vi "Send Perform Action.vi"(4 "Timeout":i32=1000, 6 "DataSocket Reply URL":string, 7 "Message Priority (Normal)":T1=enum."Normal", 8 "error in (no error)":errorcluster, 9 "Input":variant, 10 "Task-Point Ident":string, 11 "Message Enqueuer":refnum<class "Message Enqueuer.lvclass">) -> (0 "error out":errorcluster, 1 "Timeout?":bool, 2 "Reply":variant, 3 "Message Enqueuer out":refnum<class "Message Enqueuer.lvclass">)   [LabVIEW 2024, in "IMSS Target Actor.lvlib" / "Perform Action Msg.lvclass"]
doc: "This VI sends the message to an actor."
uses:
  Perform Action Msg.lvclass
  <vilib>/ActorFramework/Message Enqueuer/Message Enqueuer.lvclass
  <vilib>/ActorFramework/Message Enqueuer/Message Priority.ctl
  Perform Action Msg.lvclass/Perform Action Msg.ctl
  Reply-Msg-DataSocket/Reply Msg DataSocket/Reply Msg DataSocket.lvclass
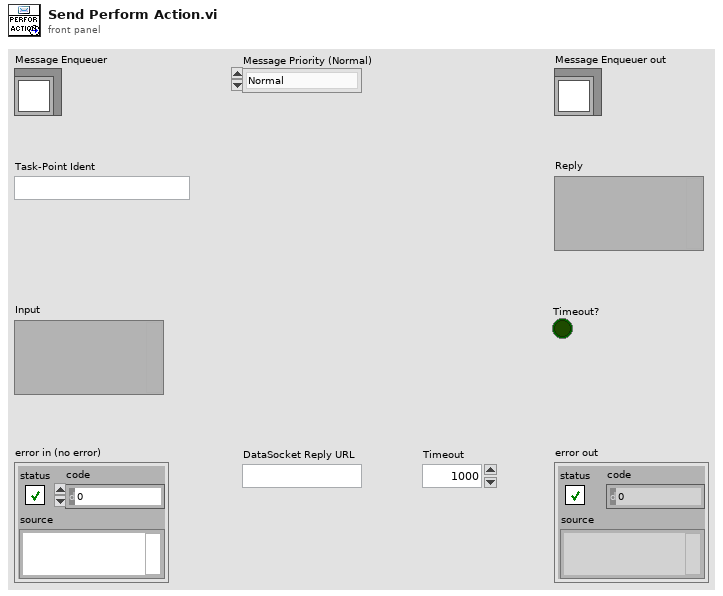
[diagram p1: front panel]
types:
  T1 = typedef "Actor Framework.lvlib/Message Enqueuer.lvclass/Message Priority.ctl" = enum16{"Low", "Normal", "High"}
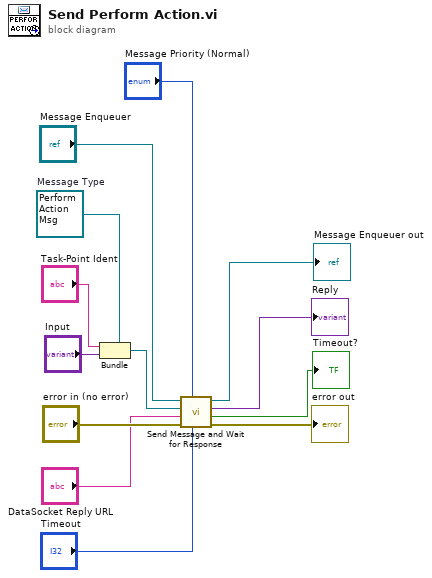
[diagram p0: block diagram]
diagram:
  w13 = refnum<class "Perform Action Msg.lvclass"> refnum  # Message Type
  n1 = Bundle(cluster=w13, "Task-Point Ident", "Input") -> (w4:refnum<class "Perform Action Msg.lvclass">)
  n2 = call "Send Message and Wait for Response.vi"("Timeout"="Timeout", "Message Priority (Normal)"="Message Priority (Normal)", "error in"="error in (no error)", "DataSocket Reply URL"="DataSocket Reply URL", "Original Message"=w4, "Message Enqueuer in"="Message Enqueuer") -> ("error out"=→"error out":errorcluster, "Timeout?"=→"Timeout?":bool, "Reply"=→"Reply":variant, "Message Enqueuer out"=→"Message Enqueuer out":refnum<class "Message Enqueuer.lvclass">)  [unwired: 2 in]
